vi "write general keywords.vi"(8 "error in (no error)":errorcluster, 11 "Save Image in":refnum<class "Save Image.lvclass">) -> (0 "error out":errorcluster, 3 "Save Image out":refnum<class "Save Image.lvclass">)   [LabVIEW 2018, in "Save Image.lvclass"]
uses:
  Save Image.lvclass
  Save Image.lvclass/Save Image.ctl
  Channel/Channel.lvclass/Channel.ctl
  Simulated_CCD_Camera/Simulated_CCD_Camera.lvclass
  Channel/Channel.lvclass
panel:
  in  "Channel information":T1
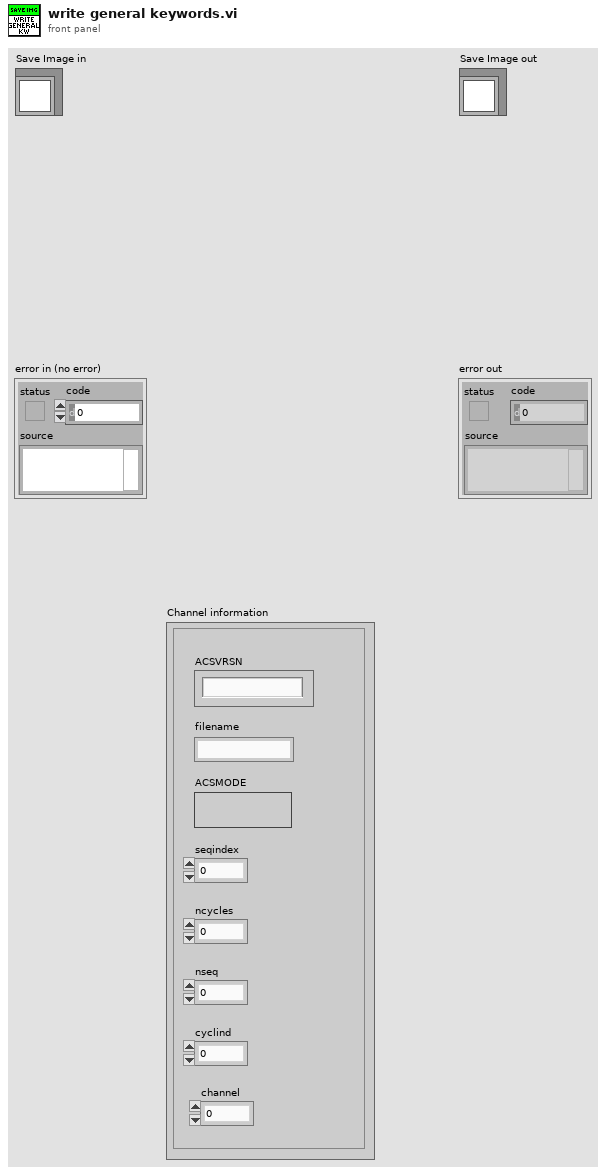
[diagram p1: front panel]
types:
  T1 = cluster{"ACSVRSN":string, "ACSMODE":bool, "filename":string, "seqindex":u16, "ncycles":u16, "nseq":u16, "cyclind":u16, "channel":u16}
  T2 = cluster{"ACS mode":bool, "Image path":path, "Remote IP":string, "Python path":path, "Communication using stream":bool}
  T3 = cluster{"CYCLES_DONE":u16, "LAST_IMAGE_NAME":string, "DISK_SPACE":u16, "FRAMES_DONE":u16, "CCD_STATUS":string, "CURRENT_TEMPERATURE":i16, "TEMPERATURE_STATUS":string, "FRAME_EXPOSURE_TIME":sgl, "ERROR":bool, "SERIAL_NUMBER":u16, "ACQUIRING":bool, "IMAGE_INDEX":u32, "SEQS_DONE":u16}
  T4 = cluster{"COOLER_POWER_STATUS":u16, "TEMP":i32, "EXPTIME":dbl, "#FRAMES":u32, "#CYCLES":u32, "#SEQS":u32, "WAVEPLATE_POS":u16}
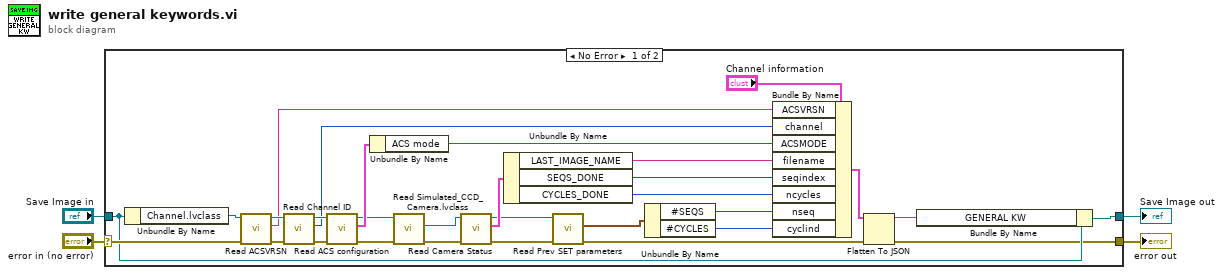
[diagram p0: block diagram]
diagram:
  n1 = case shown="No Error" "error in (no error)" {
    selector: "error in (no error)" -> [w25 w36]
    tunnel: [w8 w36] -> w3
    tunnel: [w5 w35] -> w1
    tunnel: "Save Image in" -> [w10 w35]
    frame No Error {
      n2 = Unbundle By Name(w10) -> ("Channel.lvclass"=w29:refnum<class "Channel.lvclass">)
      n3 = call "Read ACSVRSN.vi"("error in (no error)"=w25, "Channel in"=w29) -> ("error out"=w27:errorcluster, "ACSVRSN"=w26:string, "Channel out"=w28:refnum<class "Channel.lvclass">)  [unwired: 7 in]
      n4 = call-dynamic "Read Channel ID.vi"("error in (no error)"=w27, "Channel in"=w28) -> ("error out"=w32:errorcluster, "Channel ID"=w30:u8, "Channel out"=w31:refnum<class "Channel.lvclass">)  [unwired: 7 in]
      n5 = call-dynamic "Read ACS configuration.vi"("error in (no error)"=w32, "Channel in"=w31) -> ("error out"=w24:errorcluster, "ACS configuration"=w34:T2, "Channel out"=w23:refnum<class "Channel.lvclass">)  [unwired: 7 in]
      n6 = Unbundle By Name(w34) -> ("ACS mode"=w33:bool)
      n7 = call "Read Simulated_CCD_Camera.lvclass.vi"("error in (no error)"=w24, "Channel in"=w23) -> ("error out"=w21:errorcluster, "Simulated_CCD_Camera.lvclass"=w22:refnum<class "Simulated_CCD_Camera.lvclass">)  [unwired: 7 in, 1 out]
      n8 = call "Read Camera Status.vi"("error in (no error)"=w21, "CCDCamera in"=w22) -> ("error out"=w20:errorcluster, "Camera Status"=w19:T3, "CCDCamera out"=w12:refnum<class "Simulated_CCD_Camera.lvclass">)  [unwired: 7 in]
      n9 = Unbundle By Name(w19) -> ("LAST_IMAGE_NAME"=w18:string, "SEQS_DONE"=w17:u16, "CYCLES_DONE"=w16:u16)
      n10 = call-dynamic "Read Prev SET parameters.vi"("error in (no error)"=w20, "Simulated_CCD_Camera in"=w12) -> ("error out"=w9:errorcluster, "Prev SET parameters"=w15:T4)  [unwired: 7 in, 1 out]
      n11 = Unbundle By Name(w15) -> ("#SEQS"=w14:u32, "#CYCLES"=w13:u32)
      n12 = Bundle By Name(cluster="Channel information", "ACSVRSN"=w26, "channel"=w30, "ACSMODE"=w33, "filename"=w18, "seqindex"=w17, "ncycles"=w16, "nseq"=w14, "cyclind"=w13) -> (w6:T1)
      n13 = Flatten To JSON(anything=w6, error in (no error)=w9) -> (JSON string=w7:string, 11:w8:errorcluster)  [unwired: 1 in]
      n14 = Bundle By Name(cluster=w10, "GENERAL KW"=w7) -> (w5:refnum<class "Save Image.lvclass">)
    }
    frame Error {
    }
  }
  "error out" <- w3
  "Save Image out" <- w1
